vi "CAN KommTEST.vi"() -> ()   [LabVIEW 2020, in "CAN Interface.lvlib"]
uses:
  CAN Interface.lvlib
  <vilib>/xnet/xnet.llb/XNET Frame CAN.ctl
  <vilib>/xnet/xnet.llb/XNET Frame Type CAN.ctl
  <vilib>/xnet/xnet.llb/XNET Create Session (Frame Output Stream).vi
  <vilib>/xnet/xnet.llb/XNET Write (Frame CAN).vi
  <resource>/objmgr/xnet.rc
  <vilib>/xnet/xnet.llb/XNET Create Session (Frame Output Single-point).vi
panel:
  in  "Frame-ID":u32=900
  in  "Zyklus":u32=500
  out "data":T1[](array[typedef])=[{"timestamp"=timestamp(0 s since 1904-01-01), "payload"=[0, 2, 3, 4, 5, 6, 7, 8], "identifier"=2, "type"=0, "extended?"=FALSE, "echo?"=FALSE}, {"timestamp"=timestamp(0 s since 1904-01-01), "payload"=[0, 1, 2, 3, 4, 5, 6, 7], "identifier"=3, "type"=0, "extended?"=FALSE, "echo?"=FALSE}] {"payload" format="%x"; "timestamp" format="%<%.7X\n%x>T"; "type" items=["CAN Data"=0, "CAN Remote"=1, "CAN Bus Error"=2, "CAN 2.0 Data"=8, "CAN FD Data"=16, "CAN FD+BRS Data"=24, "J1939 Data"=192, "Delay"=224, "Log Trigger"=225, "Start Trigger"=226]; "identifier" format="%x"}
  out "error out":errorcluster
  in  "stop":bool
  in  "Interface Baud Rate":u32=250000
  in  "CAN Cluster":refnum<k21>="06X-52T2_171214"
  in  "Select Interface":refnum<k21>="CAN1"
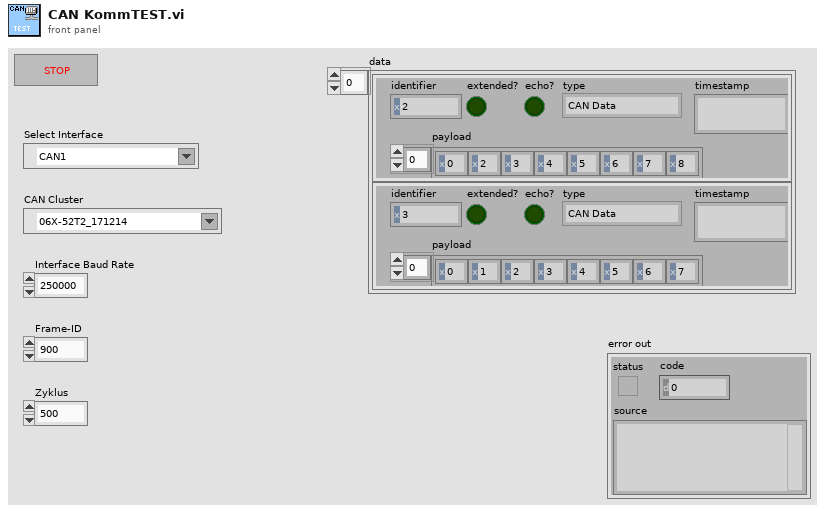
[diagram p1: front panel]
types:
  T1 = typedef "XNET Frame CAN.ctl" = cluster{"timestamp":timestamp, "payload":u8[], "identifier":u32, "type":T2, "extended?":bool, "echo?":bool}
  T2 = typedef "XNET Frame Type CAN.ctl" = u8
  T3 = enum16{"big-endian, network order", "native, host order", "little-endian"}
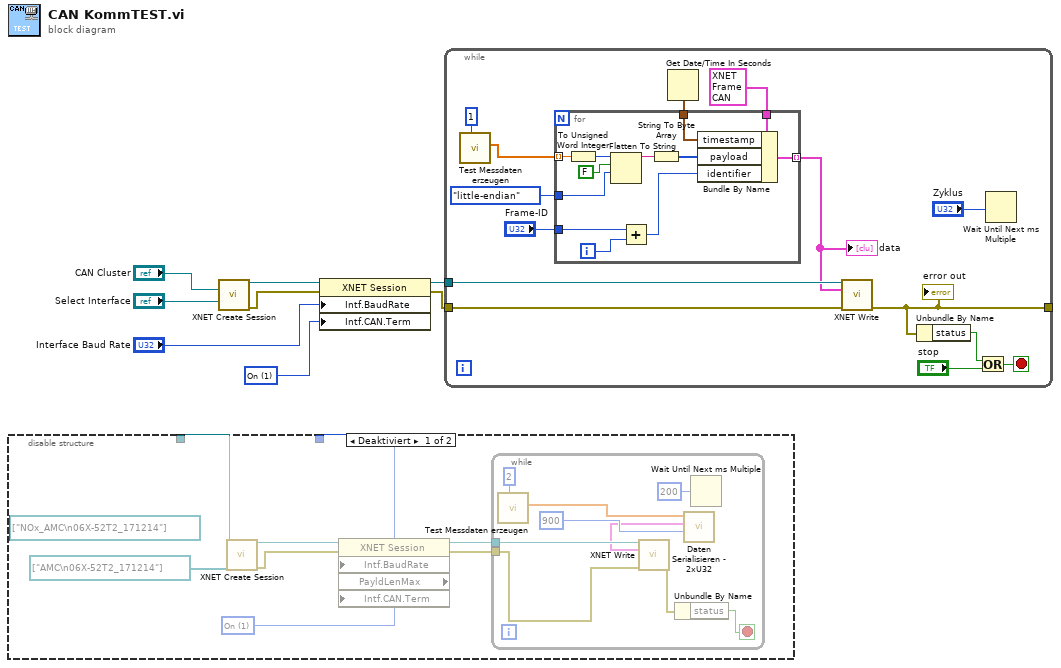
[diagram p0: block diagram]
diagram:
  w1 = u32 1 items=["Off", "On"] ("Interface:CAN:Termination")
  n1 = disable-structure shown="Deaktiviert" {
    disable-tunnel: _ -> [w16 _]
    disable-tunnel: _ -> [w15 _]
    frame Disabled {
      w9 = u32 1 items=["Off", "On"] ("Interface:CAN:Termination")
      (unwired) refnum<k21>[] ["NOx_AMC\n06X-52T2_171214"] ("signal list")
      n2 = call-poly <vilib>:"XNET Create Session.vi"("frame list"=refnum<k21>[] ["AMC\n06X-52T2_171214"], "interface"=w16) -> ("session out"=w14:refnum<k21>, "error out"=w13:errorcluster)  [unwired: 12 in]
      n3 = property class="XNET Session" props=["Intf.BaudRate", "PayldLenMax", "Intf.CAN.Term"](reference=w14, error in=w13, "Intf.BaudRate"=w15, "Intf.CAN.Term"=w9) -> (reference out=w12:refnum<k21>, error out=w11:errorcluster)  [unwired: 1 out]
      n4 = while {
        tunnel: w12 -> [w25]
        tunnel: w11 -> [w24]
        stop <- w22 stop-if-true
        n5 = call "Test Messdaten erzeugen.vi"("Anzahl Werte"=2) -> ("Messdaten"=w20:sgl[])  [unwired: 10 in]
        n6 = call "Daten Serialisieren - 2xU32.vi"("Frame-ID"=u32 900 ("identifier"), "Messdaten"=w20) -> ("data"=w17:T1[])  [unwired: 9 in]
        n7 = call-poly <vilib>:"XNET Write.vi"("session in"=w25, "data"=w17, "error in (no error)"=w24) -> ("error out"=w23:errorcluster)  [unwired: 12 out]
        n8 = Unbundle By Name(w23) -> ("status"=w22:bool)
        n9 = Wait Until Next ms Multiple(millisecond multiple=u32 200 ("milliseconds to wait")) -> ()  [unwired: 1 out]
      }
    }
    frame Enabled {
    }
  }
  n10 = call-poly <vilib>:"XNET Create Session.vi"("cluster (:memory:)"="CAN Cluster", "interface"="Select Interface") -> ("session out"=w5:refnum<k21>, "error out"=w4:errorcluster)  [unwired: 12 in]
  n11 = property class="XNET Session"(reference=w5, error in=w4, "Intf.BaudRate"="Interface Baud Rate", "Intf.CAN.Term"=w1) -> (reference out=w2:refnum<k21>, error out=w3:errorcluster)
  n12 = while {
    tunnel: w2 -> [w36]
    tunnel: w3 -> [w35]
    tunnel: [w34] -> _
    stop <- w38 stop-if-true
    n13 = call "Test Messdaten erzeugen.vi"("Anzahl Werte"=1) -> ("Messdaten"=w28:sgl[])  [unwired: 10 in]
    n14 = Get Date/Time In Seconds() -> (seconds since 1Jan1904=w29:timestamp)
    n15 = for {
      tunnel: w28 -> [w41] mode=indexing
      tunnel: T3."little-endian" ("Byte-Reihenfolge (0:Big-Endian, Netzwerkreihenfolge)") -> [w50]
      tunnel: T1 {"timestamp"=timestamp(0 s since 1904-01-01), "payload"=[0, 2, 3, 4, 5, 6, 7, 8], "identifier"=2, "type"=0, "extended?"=FALSE, "echo?"=FALSE} ("CAN frame") -> [w48]
      tunnel: "Frame-ID" -> [w45]
      tunnel: w29 -> [w43]
      tunnel: [w42] -> w27 mode=indexing
      i -> [w46]
      n16 = To Unsigned Word Integer(number=w41) -> (unsigned 16bit integer=w40:u16)
      n17 = Flatten To String(anything=w40, prepend array or string size? (T)=FALSE ("Array- oder String-Größe voranstellen? (T)"), byte order (0:big-endian, network order)=w50) -> (data string=w51:string)  [unwired: 1 in, 2 out]
      n18 = Add(x=w45, y=w46) -> (x+y=w44:u32)
      n19 = String To Byte Array(string=w51) -> (unsigned byte array=w47:u8[])
      n20 = Bundle By Name(cluster=w48, "timestamp"=w43, "payload"=w47, "identifier"=w44) -> (w42:T1)
    }
    "data" <- w27
    n21 = call-poly <vilib>:"XNET Write.vi"("session in"=w36, "data"=w27, "error in (no error)"=w35) -> ("error out"=w34:errorcluster)  [unwired: 12 out]
    "error out" <- w34
    n22 = Unbundle By Name(w34) -> ("status"=w37:bool)
    n23 = Or(x=w37, y="stop") -> (x .or. y?=w38:bool)
    n24 = Wait Until Next ms Multiple(millisecond multiple="Zyklus") -> ()  [unwired: 1 out]
  }
